vi "PolarizationInit.vi"(2 "error IO":errorcluster caption="error in") -> (0 "error IO 2":errorcluster caption="error out")   [LabVIEW 2018]
panel:
  # "初始化偏振控制器"
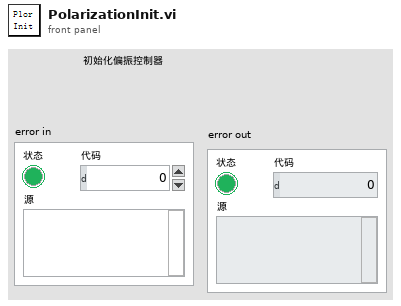
[diagram p1: front panel]
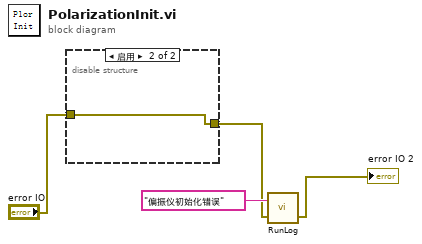
[diagram p0: block diagram]
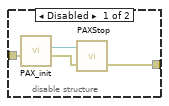
[diagram p2: hidden frame]
diagram:
  n1 = disable-structure shown="启用" {
    disable-tunnel: "error IO" -> [w8 w9]
    disable-tunnel: [w5 w9] -> w1
    frame Disabled {
      n2 = call "PAX_init.vi"("Error In"=w8) -> ("error out"=w6:errorcluster, "偏振测量仪VISA"=w7:refnum<visa-resource-name>)  [unwired: 9 in]
      n3 = call "PAXStop.vi"("error in"=w6, "VISA 输入"=w7) -> ("error out"=w5:errorcluster)  [unwired: 1 in]
    }
    frame Enabled {
    }
  }
  n4 = call "RunLog.vi"("error in"=w1, "Message"="偏振仪初始化错误") -> ("error out"=→"error IO 2":errorcluster)  [unwired: 1 in]
